vi "Open Instrument.vi"(8 "error in (no error)":errorcluster, 11 "Instrument.Oxford1820 in":refnum<class "Instrument.OxfordVRM.lvclass">) -> (0 "error out":errorcluster, 3 "Instrument.Oxford1820 out":refnum<class "Instrument.OxfordVRM.lvclass">)   [LabVIEW 2016, in "Instrument.OxfordVRM.lvclass"]
uses:
  Instrument.OxfordVRM.lvclass
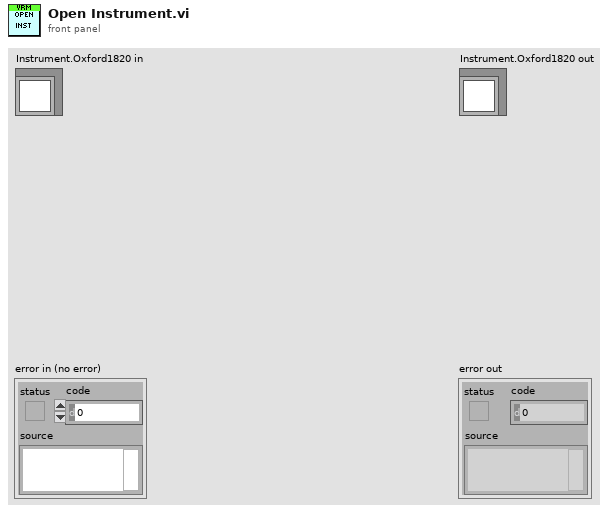
[diagram p1: front panel]
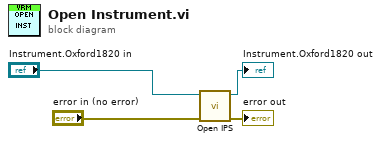
[diagram p0: block diagram]
diagram:
  n1 = call "Open IPS.vi"("error in (no error)"="error in (no error)", "Instrument.OxfordVRM in"="Instrument.Oxford1820 in") -> ("error out"=→"error out":errorcluster, "Instrument.OxfordVRM out"=→"Instrument.Oxford1820 out":refnum<class "Instrument.OxfordVRM.lvclass">)  [unwired: 8 in]
